vi "compression pin map test.vi"() -> ()   [LabVIEW 2021]
uses:
  Classes/Controller/I-O/I-O.lvclass
  Classes/Controller/Controller.lvclass
panel:
  in  "stop":bool
  out "Compression":bool=TRUE
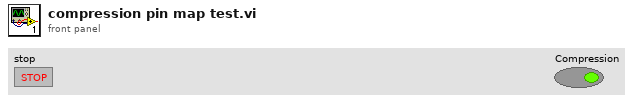
[diagram p1: front panel]
types:
  T1 = typedef "Controller.lvclass/Controllers.ctl" = cluster{"I-O.lvclass":refnum<class "I-O.lvclass">, "Gantry":refnum<k24>, "Dispenser":refnum<visa-resource-name>}
  T2 = typedef "I-O.lvclass/Pin Map.ctl" = cluster{"Region Valves":i32[], "Extra Valves":dbl[][][], "Tool Primary Valve":i32, "Tool Secondary Valve":i32, "Region Sensors":i32[], "Extra Sensors":dbl[][][], "Tool Primary Sensor":dbl, "Tool Secondary Sensor":dbl, "Compression Sensor":dbl, "5V":i32, "Dispenser Sensor":dbl}
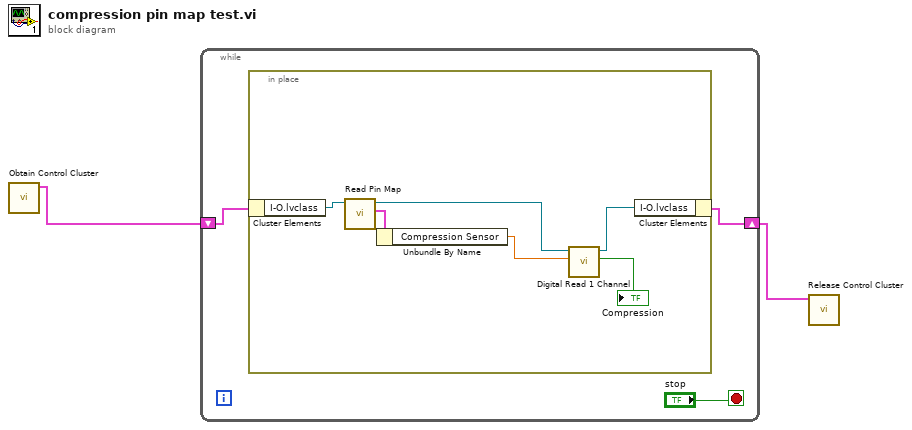
[diagram p0: block diagram]
diagram:
  n1 = call "Obtain Control Cluster.vi"() -> ("Control Out"=w2:T1)  [unwired: 11 in]
  n2 = while {
    shift-right: [w4] -> w1
    shift-left: w2 -> [w5]
    stop <- "stop" stop-if-true
    n3 = in-place {
      n4 = in-place-cluster #1(w5) -> ("I-O.lvclass"=w11:refnum<class "I-O.lvclass">)
      n5 = call-dynamic "Read Pin Map.vi"("I-O in"=w11) -> ("Pin Map 2"=w10:T2, "I-O out"=w8:refnum<class "I-O.lvclass">)  [unwired: 8 in, 1 out]
      n6 = Unbundle By Name(w10) -> ("Compression Sensor"=w9:dbl)
      n7 = call-dynamic "Digital Read 1 Channel.vi"("Read"=w9, "I-O in"=w8) -> ("Value"=→"Compression":bool, "I-O out"=w7:refnum<class "I-O.lvclass">)  [unwired: 7 in, 1 out]
      n8 = in-place-cluster #1("I-O.lvclass"=w7) -> (w4:T1)
    }
  }
  n9 = call "Release Control Cluster.vi"("output cluster"=w1) -> ()  [unwired: 11 in]
